vi "Folgen zu Überholen.vi"(8 "hinten links":dbl, 9 "hinten rechts":dbl, 10 "vorne links":dbl, 11 "vorne rechts":dbl) -> (3 "Überholstrecke?":bool)   [LabVIEW 2016]
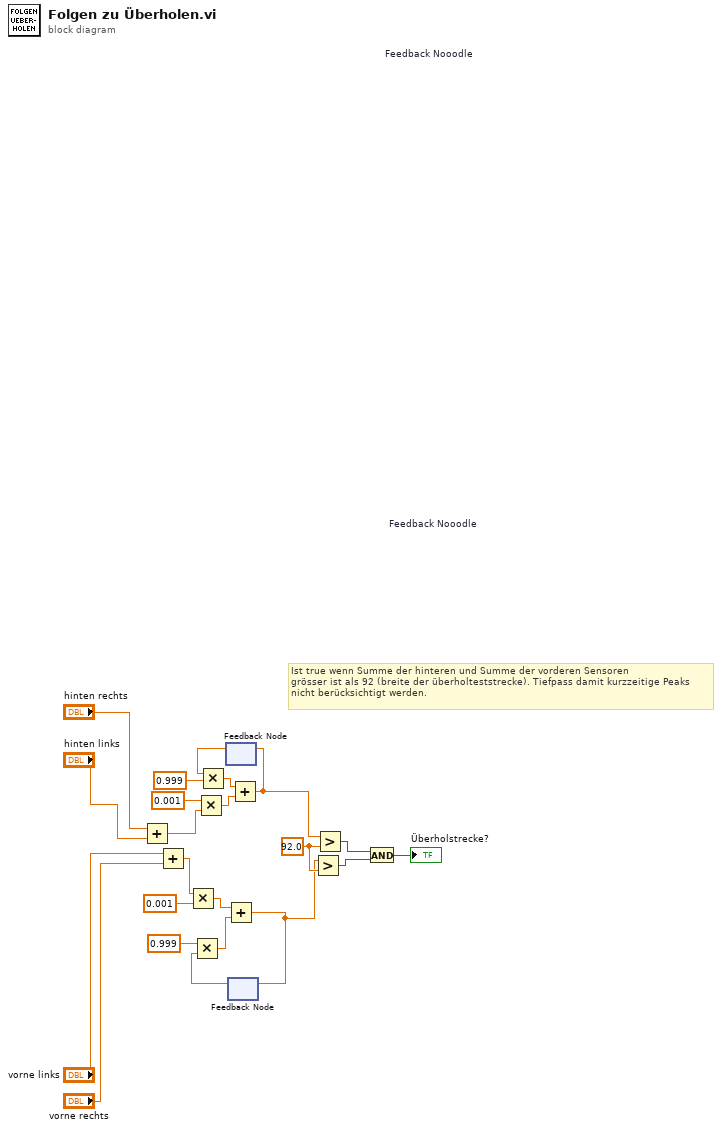
[diagram p0: block diagram]
diagram:
  w18 = 92.0 ("y")
  # "Ist true wenn Summe der hinteren und Summe der vorderen Sensoren\ngrösser ist als 92 (breite der überholteststrecke). Tiefpass damit kurzzeitige Peaks\nnicht berücksichtigt werden."
  n1 = Add(x="hinten rechts", y="hinten links") -> (x+y=w14:dbl)
  n2 = Add(x="vorne links", y="vorne rechts") -> (x+y=w7:dbl)
  n3 = Multiply(x=w7, y=0.001) -> (x*y=w5:dbl)
  n4 = Multiply(x=0.001, y=w14) -> (x*y=w9:dbl)
  n5 = feedback #1 "Feedback Nooodle"() -> (w12:dbl)  [unwired: 1 in]
  n6 = Multiply(x=w12, y=0.999) -> (x*y=w10:dbl)
  n7 = feedback #2 "Feedback Nooodle"() -> (w4:dbl)  [unwired: 1 in]
  n8 = Multiply(x=0.999, y=w4) -> (x*y=w2:dbl)
  n9 = Add(x=w5, y=w2) -> (x+y=w1:dbl)
  n10 = feedback-in #2(w1) -> ()
  n11 = Add(x=w10, y=w9) -> (x+y=w8:dbl)
  n12 = feedback-in #1(w8) -> ()
  n13 = Greater?(x=w1, y=w18) -> (0:w16:bool)
  n14 = Greater?(x=w8, y=w18) -> (0:w17:bool)
  n15 = And(x=w17, y=w16) -> (x .and. y?=→"Überholstrecke?":bool)
